vi "decodeInt.vi"(8 "error in (no error)":errorcluster, 10 "ByteArray":u8[](array[numeric])=[0, 255, 255] format="%.0x") -> (0 "error out":errorcluster, 1 "uint":i64, 2 "variant":variant, 3 "RemainingBytes":u8[](array[numeric]), 5 "Type":string)   [LabVIEW 2020, in "MsgPack.lvlib"]
uses:
  MsgPack.lvlib
  <vilib>/Utility/error.llb/Error Cluster From Error Code.vi
  <vilib>/ErrorRing/Error Ring.xnode
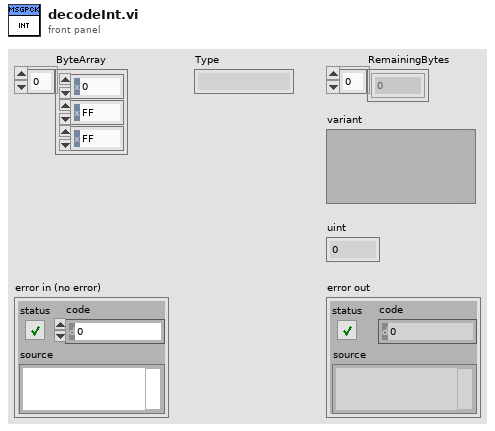
[diagram p1: front panel]
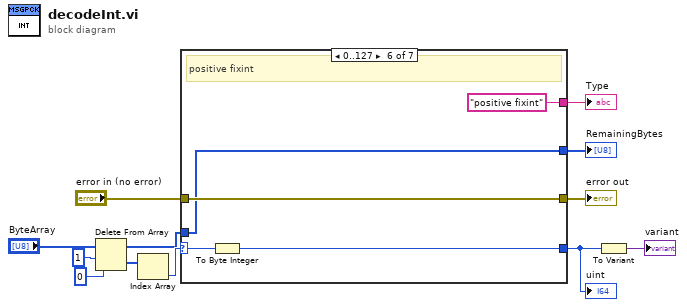
[diagram p0: block diagram]
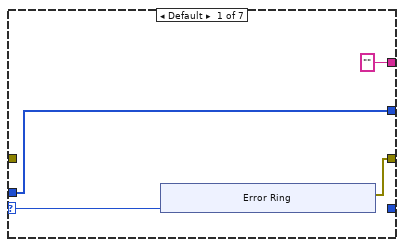
[diagram p2: hidden frame]
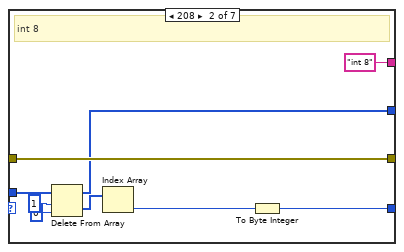
[diagram p3: hidden frame]
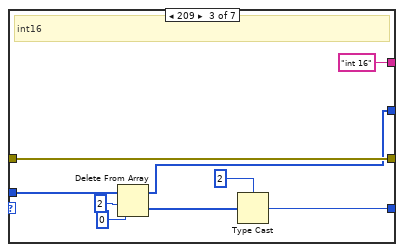
[diagram p4: hidden frame]
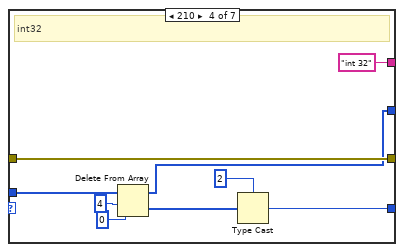
[diagram p5: hidden frame]
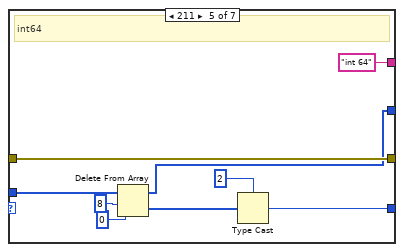
[diagram p6: hidden frame]
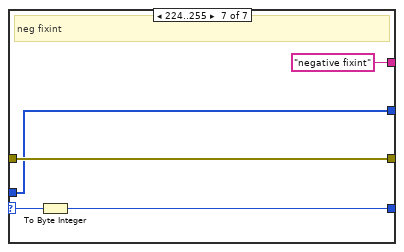
[diagram p7: hidden frame]
diagram:
  n1 = Delete From Array(array="ByteArray", length=1, index=0) -> (deleted portion=w2:u8[], array with subset deleted=w3:u8[])
  n2 = Index Array(array=w2) -> (element=w9:u8)  [unwired: 1 in]
  n3 = case shown="0..127" w9 {
    selector: w9 -> [w14 _ _ _ _ w64 w66]
    tunnel: [w15 w32 w41 w50 w59 w61 w67] -> w11
    tunnel: "error in (no error)" -> [_ w32 w41 w50 w59 w61 w67]
    tunnel: ["" "int 8" "int 16" "int 32" "int 64" "positive fixint" "negative fixint"] -> w8
    tunnel: [_ w30 w39 w48 w57 w63 w69] -> w7
    tunnel: w3 -> [w13 w27 w37 w46 w55 w60 w65]
    tunnel: [w13 w25 w35 w45 w52 w60 w65] -> w6
    frame Default {
      n4 = xnode "Error Ring"("parameter 0"=w14) -> ("error out"=w15:errorcluster)
    }
    frame 208 {
      # "int 8"
      n5 = Delete From Array(array=w27, length=1, index=0) -> (deleted portion=w26:u8[], array with subset deleted=w25:u8[])
      n6 = Index Array(array=w26) -> (element=w29:u8)  [unwired: 1 in]
      n7 = To Byte Integer(number=w29) -> (8bit integer=w30:i8)
    }
    frame 209 {
      # "int16"
      n8 = Delete From Array(array=w37, length=2, index=0) -> (deleted portion=w34:u8[], array with subset deleted=w35:u8[])
      n9 = Type Cast(type=i16 2 ("length"), x=w34) -> (*(type *) &x=w39:i16)
    }
    frame 210 {
      # "int32"
      n10 = Delete From Array(array=w46, length=4, index=0) -> (deleted portion=w44:u8[], array with subset deleted=w45:u8[])
      n11 = Type Cast(type=2 ("length"), x=w44) -> (*(type *) &x=w48:i32)
    }
    frame 211 {
      # "int64"
      n12 = Delete From Array(array=w55, length=8, index=0) -> (deleted portion=w53:u8[], array with subset deleted=w52:u8[])
      n13 = Type Cast(type=i64 2 ("length"), x=w53) -> (*(type *) &x=w57:i64)
    }
    frame 0..127 {
      # "positive fixint"
      n14 = To Byte Integer(number=w64) -> (8bit integer=w63:i8)
    }
    frame 224..255 {
      # "neg fixint"
      n15 = To Byte Integer(number=w66) -> (8bit integer=w69:i8)
    }
  }
  "error out" <- w11
  "Type" <- w8
  "uint" <- w7
  "RemainingBytes" <- w6
  n16 = To Variant(anything=w7) -> (Variant=→"variant":variant)
